vi "iHR550 Convert Axis v10.5.0.vi"(1 "CCD Area Format":T1, 2 "iHR Current Values":T3={"iHR 550 Front Entrance"=0.0, "iHR550 Side Exit"=0.0, "iHR550 Wavelength"=897.9988, "iHR550 Exit Mirror"=2, "iHR550 Grating"="1", "Grating Index"=1} {"iHR550 Exit Mirror" items=["EntranceMirror", "ExitMirror", "Front", "Side"]}) -> (0 "Wavelengths (nm)":dbl[](array[numeric]))   [LabVIEW 2010]
uses:
  TypeDefs/iHR Current Values.ctl
  TypeDefs/iHR Instrument Parameters.ctl
  Symphony/TypeDefs/Symphony Area Format.ctl
panel:
  out "Tabellen-String":string
  out "l_p (nm)":dbl
  out "beta_lp (rad)":dbl
  out "H_Blp (mm)":dbl
  out "P_c":dbl
  out "beta_H (rad)":dbl
  out "beta_lc (rad)":dbl
  in  "Diffraction Order":i8=1
  in  "Grooves (1/mm)":i16[](array[numeric])=[1800, 600, 150]
  out "alpha_lc (rad)":dbl
  out "H_Blc (mm)":dbl
  out "L_H (mm)":dbl
  out "Inclination Angle (rad)":dbl
  out "Ebert Angle (rad)":dbl
  out "Pixel Width (mm)":dbl
  in  "iHR Instrument Parameters":T2={"Focal In (mm)"=546.0, "Focal Out (mm)"=568.72, "Pixel Width (µm)"=13.5, "Pixel Count"=2048, "Ebert Angle (°)"=6.498, "Inclination Angle (°)"=-2.35}
  # "pixel count could\nalso be read from CCD"
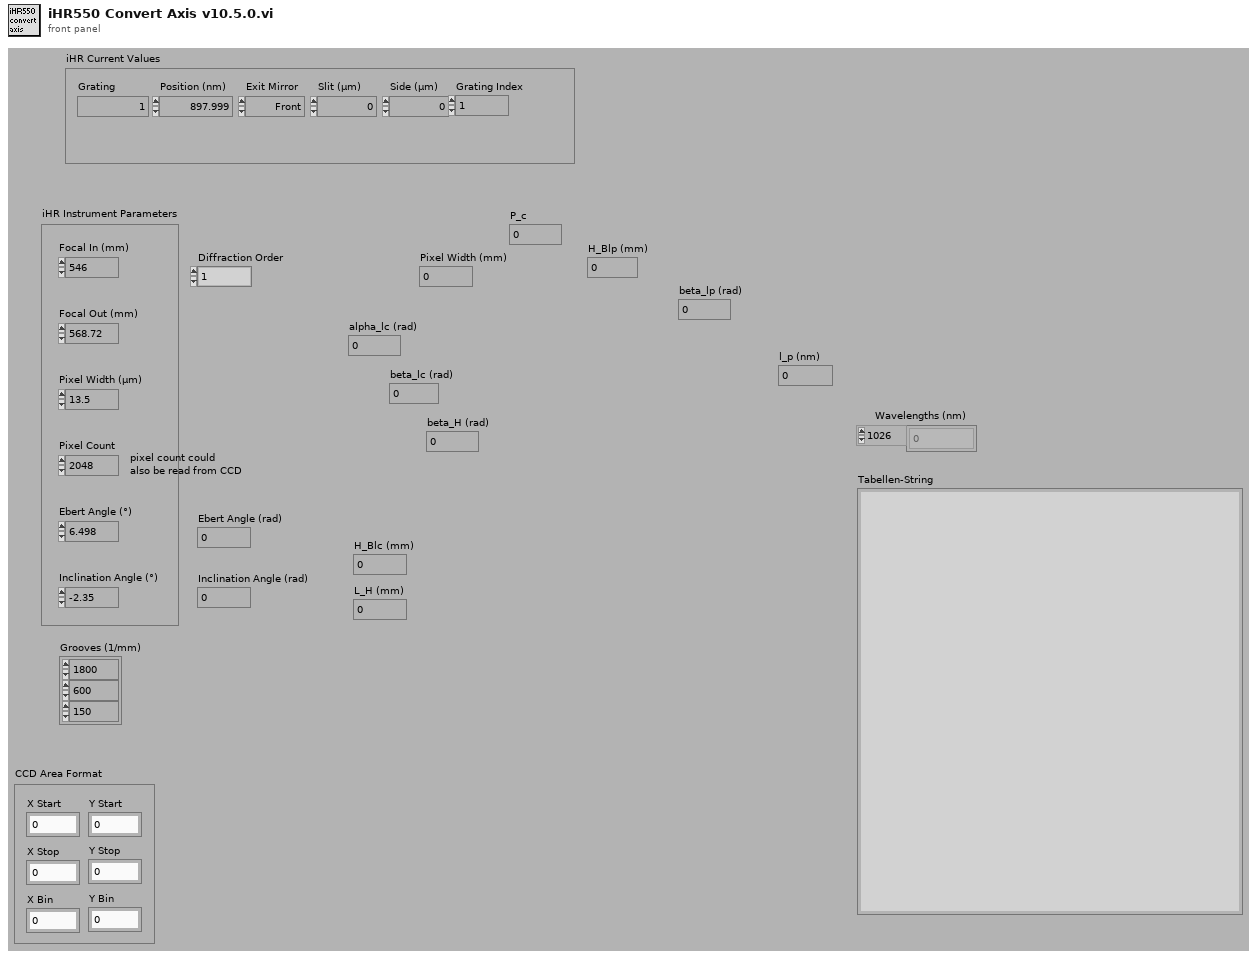
[diagram p1: front panel]
types:
  T1 = typedef "Symphony Area Format.ctl" = cluster{"XStart":i32, "YStart":i32, "XStop":i32, "YStop":i32, "XBin":i32, "YBin":i32}
  T2 = typedef "iHR Instrument Parameters.ctl" = cluster{"Focal In (mm)":dbl, "Focal Out (mm)":dbl, "Pixel Width (µm)":dbl, "Pixel Count":i16, "Ebert Angle (°)":dbl, "Inclination Angle (°)":dbl}
  T3 = typedef "iHR Current Values.ctl" = cluster{"iHR 550 Front Entrance":dbl, "iHR550 Side Exit":dbl, "iHR550 Wavelength":dbl, "iHR550 Exit Mirror":i32, "iHR550 Grating":string, "Grating Index":i32}
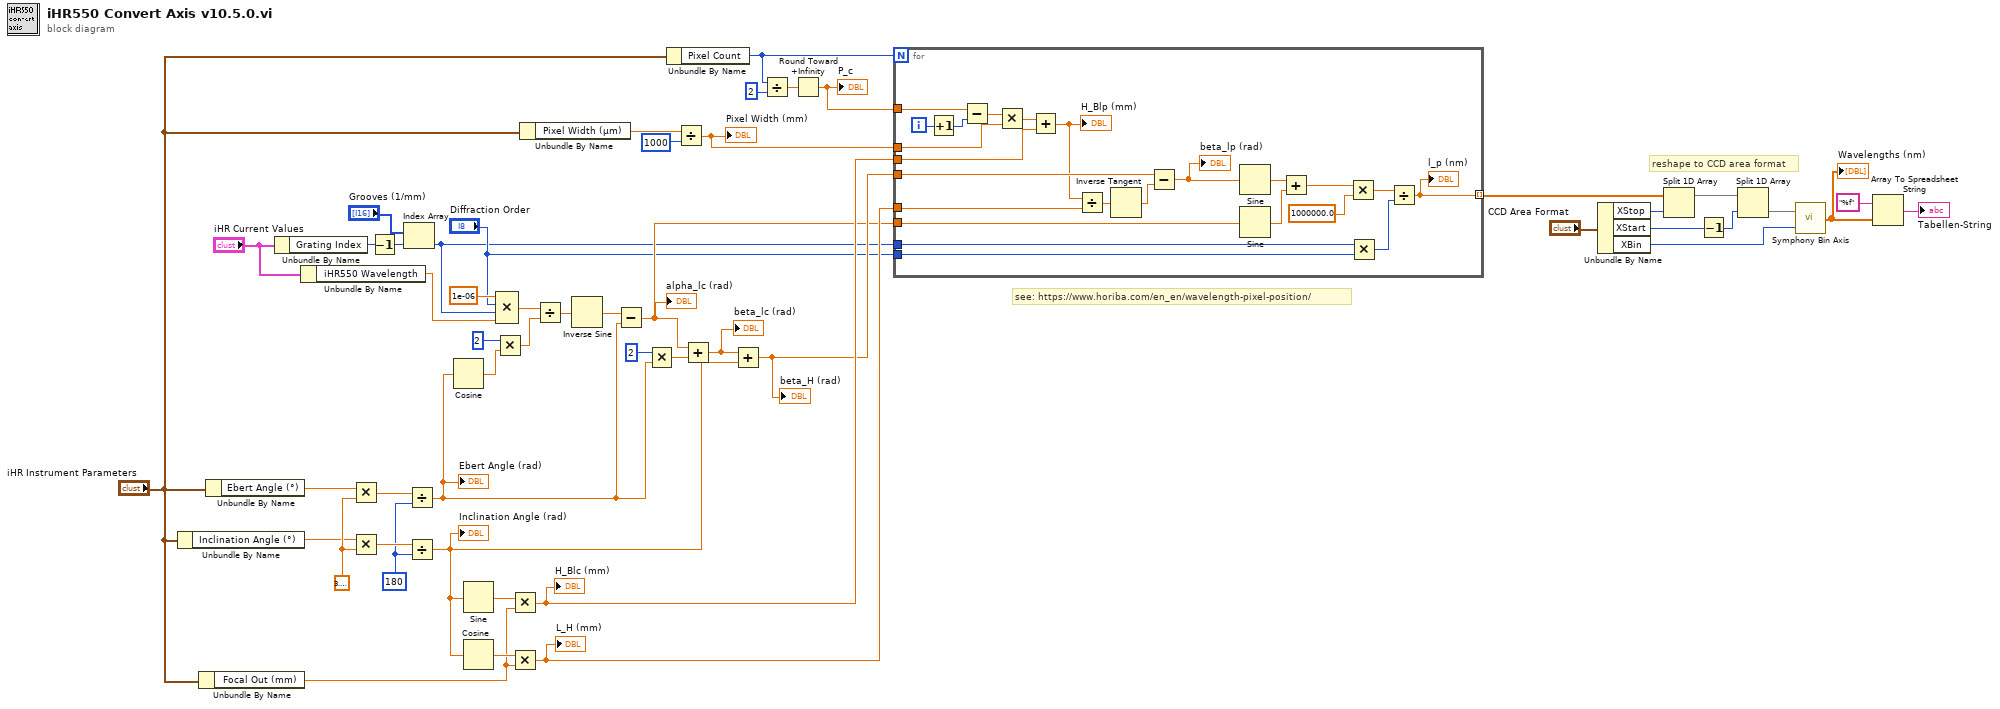
[diagram p0: block diagram]
diagram:
  w48 = i16 180 ("y")
  w50 = 3.141592653589793
  # "reshape to CCD area format"
  # "see: https://www.horiba.com/en_en/wavelength-pixel-position/"
  n1 = Unbundle By Name("iHR Instrument Parameters") -> ("Inclination Angle (°)"=w44:dbl)
  n2 = Unbundle By Name("iHR Instrument Parameters") -> ("Focal Out (mm)"=w40:dbl)
  n3 = Unbundle By Name("iHR Instrument Parameters") -> ("Ebert Angle (°)"=w45:dbl)
  n4 = Unbundle By Name("iHR Current Values") -> ("Grating Index"=w33:i32)
  n5 = Unbundle By Name("iHR Current Values") -> ("iHR550 Wavelength"=w28:dbl)
  n6 = Multiply(x=w45, y=w50) -> (x*y=w51:dbl)
  n7 = Multiply(x=w44, y=w50) -> (x*y=w49:dbl)
  n8 = Decrement(x=w33) -> (x-1=w32:i32)
  n9 = Index Array(array="Grooves (1/mm)", index=w32) -> (element=w12:i16)
  n10 = Divide(x=w51, y=w48) -> (x/y=w25:dbl)
  "Ebert Angle (rad)" <- w25
  n11 = Divide(x=w49, y=w48) -> (x/y=w23:dbl)
  "Inclination Angle (rad)" <- w23
  n12 = Cosine(x=w25) -> (cos(x)=w35:dbl)
  n13 = Sine(x=w23) -> (sin(x)=w41:dbl)
  n14 = Cosine(x=w23) -> (cos(x)=w42:dbl)
  n15 = Multiply(x=i8 2, y=w35) -> (x*y=w37:dbl)
  n16 = Compound Arithmetic op=MULTIPLY(1e-06 ("value"), "Diffraction Order", w12, w28) -> (w30:dbl)
  n17 = Multiply(x=w41, y=w40) -> (x*y=w22:dbl)
  "H_Blc (mm)" <- w22
  n18 = Multiply(x=w42, y=w40) -> (x*y=w15:dbl)
  "L_H (mm)" <- w15
  n19 = Unbundle By Name("iHR Instrument Parameters") -> ("Pixel Width (µm)"=w46:dbl)
  n20 = Divide(x=w30, y=w37) -> (x/y=w38:dbl)
  n21 = Inverse Sine(1:w38) -> (0:w39:dbl)
  n22 = Subtract(x=w39, y=w25) -> (x-y=w14:dbl)
  "alpha_lc (rad)" <- w14
  n23 = Multiply(x=i8 2, y=w25) -> (x*y=w26:dbl)
  n24 = Unbundle By Name("iHR Instrument Parameters") -> ("Pixel Count"=w21:i16)
  n25 = Divide(x=w46, y=i16 1000) -> (x/y=w17:dbl)
  "Pixel Width (mm)" <- w17
  n26 = Add(x=w14, y=w26) -> (x+y=w24:dbl)
  "beta_lc (rad)" <- w24
  n27 = Add(x=w24, y=w23) -> (x+y=w16:dbl)
  "beta_H (rad)" <- w16
  n28 = Divide(x=w21, y=i16 2) -> (x/y=w19:dbl)
  n29 = Round Toward +Infinity(x=w19) -> (ceil(x): smallest int >= x=w18:dbl)
  "P_c" <- w18
  n30 = for {
    N: w21 -> [_]
    tunnel: w22 -> [w73]
    tunnel: w18 -> [w70]
    tunnel: w17 -> [w68]
    tunnel: w16 -> [w66]
    tunnel: w15 -> [w63]
    tunnel: [w58] -> w8 mode=indexing
    tunnel: w14 -> [w56]
    tunnel: "Diffraction Order" -> [w53]
    tunnel: w12 -> [w52]
    i -> [w72]
    n31 = Increment(x=w72) -> (x+1=w71:i32)
    n32 = Subtract(x=w70, y=w71) -> (x-y=w69:dbl)
    n33 = Multiply(x=w69, y=w68) -> (x*y=w74:dbl)
    n34 = Add(x=w74, y=w73) -> (x+y=w64:dbl)
    "H_Blp (mm)" <- w64
    n35 = Divide(x=w64, y=w63) -> (x/y=w65:dbl)
    n36 = Inverse Tangent(1:w65) -> (0:w67:dbl)
    n37 = Subtract(x=w66, y=w67) -> (x-y=w57:dbl)
    "beta_lp (rad)" <- w57
    n38 = Sine(x=w57) -> (sin(x)=w55:dbl)
    n39 = Sine(x=w56) -> (sin(x)=w54:dbl)
    n40 = Add(x=w55, y=w54) -> (x+y=w61:dbl)
    n41 = Multiply(x=w61, y=1000000.0) -> (x*y=w59:dbl)
    n42 = Multiply(x=w52, y=w53) -> (x*y=w62:i16)
    n43 = Divide(x=w59, y=w62) -> (x/y=w58:dbl)
    "l_p (nm)" <- w58
  }
  n44 = Unbundle By Name("CCD Area Format") -> ("XStop"=w3:i32, "XStart"=w2:i32, "XBin"=w6:i32)
  n45 = Split 1D Array(array=w8, index=w3) -> (first subarray=w7:dbl[])  [unwired: 1 out]
  n46 = Decrement(x=w2) -> (x-1=w1:i32)
  n47 = Split 1D Array(array=w7, index=w1) -> (second subarray=w5:dbl[])  [unwired: 1 out]
  n48 = call "Symphony Bin Axis.vi"("Binning Factor"=w6, "Axis In"=w5) -> ("Axis Out"=w4:dbl[])
  "Wavelengths (nm)" <- w4
  n49 = Array To Spreadsheet String(array=w4, 3:"%f" ("Format-String")) -> (spreadsheet string=→"Tabellen-String":string)  [unwired: 1 in]
